vi "Get RPC CloseMUXChannel __Input.vi"(8 "error in (no error)":errorcluster, 11 "gRPCid in":T1) -> (0 "error out":errorcluster, 2 "Message Data":T2, 3 "gRPCid out":T1)   [LabVIEW 2019, in "ctet_mux.lvlib" / "ctet_mux.lvclass"]
uses:
  ctet_mux.lvclass
  gRPC lvSupport/Server API/typeDefs/grpcId.ctl
  RPC Messages/measurementservice_MUXCloseChannelRequest/measurementservice_MUXCloseChannelRequest_Data.ctl
  gRPC lvSupport/gprc-lvsupport.lvlib
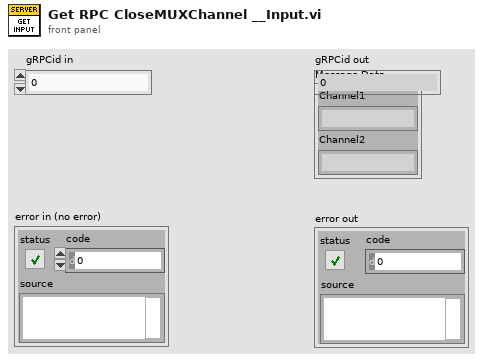
[diagram p1: front panel]
types:
  T1 = typedef "ctet_mux.lvlib/gprc-lvsupport.lvlib/grpcId.ctl" = u64
  T2 = typedef "ctet_mux.lvlib/ctet_mux.lvclass/measurementservice_MUXCloseChannelRequest_Data.ctl" = cluster{"Channel1":string, "Channel2":string}
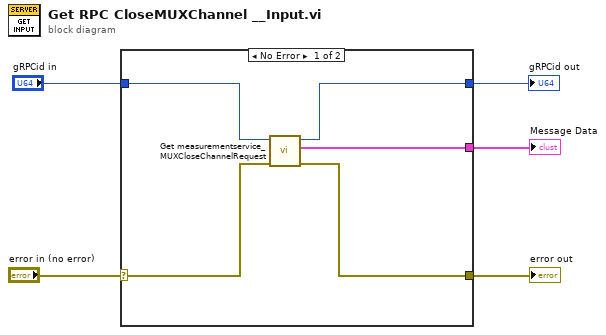
[diagram p0: block diagram]
diagram:
  n1 = case shown="No Error" "error in (no error)" {
    selector: "error in (no error)" -> [w10 w11]
    tunnel: [w9 w11] -> w4
    tunnel: "gRPCid in" -> [w8 w12]
    tunnel: [w7 _] -> w2
    tunnel: [w6 w12] -> w1
    frame No Error {
      n2 = call "Get measurementservice_MUXCloseChannelRequest.vi"("error in (no error)"=w10, "gRPCid"=w8) -> ("error out"=w9:errorcluster, "Message Data"=w7:T2, "gRPCid out"=w6:T1)  [unwired: 7 in]
    }
    frame Error {
    }
  }
  "error out" <- w4
  "Message Data" <- w2
  "gRPCid out" <- w1
